vi "VideoCapture Open_Device.vi"(8 "error in (no error)":errorcluster, 9 "apiPreference":T1 items=["CAP_ANY"=0, "CAP_VFW/CAP_V4L"=200, "CAP_FIREWIRE"=300, "CAP_QT"=500, "CAP_UNICAP"=600, "CAP_DSHOW"=700, "CAP_PVAPI"=800, "CAP_OPENNI"=900, "CAP_OPENNI_ASUS"=910, "CAP_ANDROID"=1000, "CAP_XIAPI"=1100, "CAP_AVFOUNDATION"=1200, "CAP_GIGANETIX"=1300, "CAP_MSMF"=1400, "CAP_WINRT"=1410, "CAP_INTELPERC/CAP_REALSENSE"=1500, "CAP_OPENNI2"=1600, "CAP_OPENNI2_ASUS"=1610, "CAP_OPENNI2_ASTRA"=1620, "CAP_GPHOTO2"=1700, "CAP_GSTREAMER"=1800, "CAP_FFMPEG"=1900, "CAP_IMAGES"=2000, "CAP_ARAVIS"=2100, "CAP_OPENCV_MJPEG"=2200, "CAP_INTEL_MFX"=2300, "CAP_XINE"=2400, "CAP_UEYE"=2500, "CAP_OBSENSOR"=2600], 10 "index":i32, 11 "VideoCapture in":refnum<class "VideoCapture.lvclass">) -> (0 "error out":errorcluster, 2 "Success":bool, 3 "VideoCapture out":refnum<class "VideoCapture.lvclass">)   [LabVIEW 2020, in "OpenLvVision_OpenCv.lvlib" / "VideoCapture.lvclass"]
doc: "Opens a camera for video capturing."
uses:
  VideoCapture.lvclass
  C:/Users/lukas/Downloads/OpenLvVision_OpenCv/SourceCode/LabView/OpenLvVision_OpenCv/_LvHelpers/EdvrObject/EdvrObject.lvclass
  TypeDef/VideoCaptureAPIs.ctl
  _LvHelpers/EdvrObject/EdvrObject.lvclass/EdvrObject.ctl
  OpenLvVision_OpenCv.lvlib
  _LvHelpers/EdvrObject/EdvrObject.lvclass
  Dlls/OlvOpenCvWrapper.dll
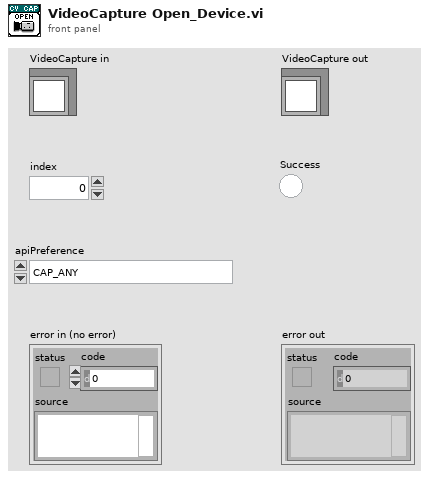
[diagram p1: front panel]
types:
  T1 = typedef "OpenLvVision_OpenCv.lvlib/VideoCaptureAPIs.ctl" = i32
  T2 = typedef "OpenLvVision_OpenCv.lvlib/EdvrObject.lvclass/Edvr.ctl" = refnum<data-value>
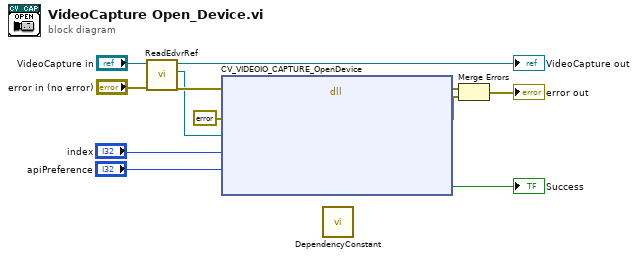
[diagram p0: block diagram]
diagram:
  n1 = call "ReadEdvrRef.vi"("error in (no error)"="error in (no error)", "EdvrObject in"="VideoCapture in") -> ("error out"=w10:errorcluster, "Edvr"=w9:T2, "EdvrObject out"=→"VideoCapture out":refnum<class "VideoCapture.lvclass">)  [unwired: 7 in]
  n2 = dll-call lib="C:/Users/lukas/Downloads/OpenLvVision_OpenCv/SourceCode/LabView/OpenLvVision_OpenCv/Dlls/OlvOpenCvWrapper.dll" fn="CV_VIDEOIO_CAPTURE_OpenDevice"(error in=w10, "Error"=errorcluster {"status"=FALSE, "code"=0, "source"=""} ("error out"), "edvrRef"=w9, "index"="index", "apiPreference"="apiPreference") -> (error out=w8:errorcluster, "Error"=w7:errorcluster, "Success"=→"Success":bool)  [unwired: 7 in, 1 out]
  n3 = call "DependencyConstant.vi"() -> ()  [unwired: 12 in]
  n4 = Merge Errors(w8, w7) -> (→"error out":errorcluster)
